vi "To Serial Form.vi"(6 "Serial Version":T1, 10 "Serializer in":refnum<class "Serializer.lvclass">, 11 "MC Data in":refnum<class "MC Data.lvclass">) -> (0 "error out":errorcluster, 2 "Serializer out":refnum<class "Serializer.lvclass">, 3 "MC Data out":refnum<class "MC Data.lvclass">)   [LabVIEW 2014, in "MC Data.lvclass"]
uses:
  MC Data.lvclass
  <vilib>/NI/AQ Character Lineator/Serializer/Serializer.lvclass
  <vilib>/NI/AQ Character Lineator/Serialization Common/Serial Version.ctl
  MC Data.lvclass/MC Data.ctl
  <vilib>/NI/AQ Character Lineator/Serializable/Insert Single.vi
  <vilib>/NI/AQ Character Lineator/Serializer/Insert Single.vi
  <vilib>/NI/AQ Character Lineator/Serializer/Read Include Default Values.vi
  Alicat Data.lvclass
  <vilib>/NI/AQ Character Lineator/Serializable/Serializable.lvclass
  <vilib>/NI/AQ Character Lineator/Serialization Common/Serialization Common.lvlib
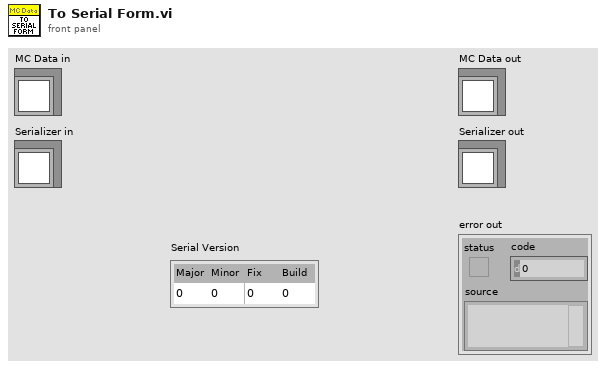
[diagram p1: front panel]
types:
  T1 = typedef "Serialization Common.lvlib/Serial Version.ctl" = cluster{"Major":u16, "Minor":u16, "Fix":u16, "Build":u16}
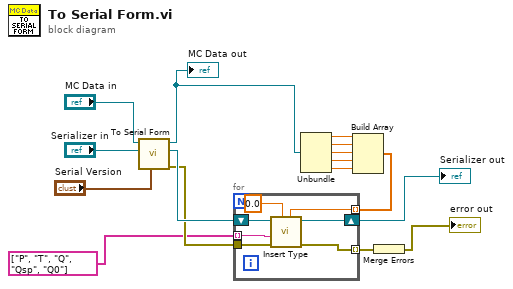
[diagram p0: block diagram]
diagram:
  n1 = call-parent "To Serial Form.vi"("Serial Version"="Serial Version", "Serializer in"="Serializer in", "Data in"="MC Data in") -> ("error out"=w5:errorcluster, "Serializer out"=w13:refnum<class "Serializer.lvclass">, "Data out"=w12:refnum<class "MC Data.lvclass">)  [unwired: 6 in]
  "MC Data out" <- w12
  n2 = Unbundle(w12) -> (w11:sgl, w10:sgl, w9:sgl, w8:sgl, w7:sgl)
  n3 = Build Array(w11, w10, w9, w8, w7) -> (w6:sgl[])
  n4 = for {
    shift-right: [w22] -> w1
    shift-left: w13 -> [w23]
    tunnel: w6 -> [w21] mode=indexing
    tunnel: w5 -> [w19]
    tunnel: [w18] -> w4 mode=indexing
    tunnel: string[] ["P", "T", "Q", "Qsp", "Q0"] -> [w17] mode=indexing
    n5 = call-poly <vilib>:"Insert Type.vi"("Double"=w21, "Default Value"=sgl 0.0, "error in (no error)"=w19, "Name"=w17, "Serializer in"=w23) -> ("error out"=w18:errorcluster, "Serializer out"=w22:refnum<class "Serializer.lvclass">)  [unwired: 5 in]
  }
  "Serializer out" <- w1
  n6 = Merge Errors(w4) -> (→"error out":errorcluster)
